vi "海洋光学光谱仪.vi"() -> ()   [LabVIEW 2018]
uses:
  <vilib>/Utility/file.llb/Write Delimited Spreadsheet (DBL).vi
  <vilib>/Utility/file.llb/Write Delimited Spreadsheet (string).vi
  Labview/SeaBreeze.lvlib
panel:
  in  "停止 2":bool
  out "当前时间":timestamp
  out "状态":string
  out "is Big Energy":bool
  out "time":string
  out "温度计":dbl(slide) scale=0.0..100.0
  out "湿度":dbl
  in  "VISA resource name":refnum<visa-resource-name>="COM3" caption="VISA资源名称"
  in  "停止":bool
  out "error_code out end":i32
  in  "count":dbl
  out "center2":dbl
  in  "baseline":dbl=2000.0 format="%#_13g"
  out "长度":i32
  out "center wavelength":dbl
  out "falling":dbl
  out "FPWM":dbl
  out "rasing":dbl
  in  "mode 触发模式为2":i32=2
  out "Type":string
  out "Grpah":cluster{"Y":dbl[], "Y":dbl[]}[](graph)
  out "Pixels":i32
  in  "integration time(us)":u32=60000
  out "Serial Number":string
  out "Found Spectrometer":string
  out "error_code out":i32
  in  "error_code":i32
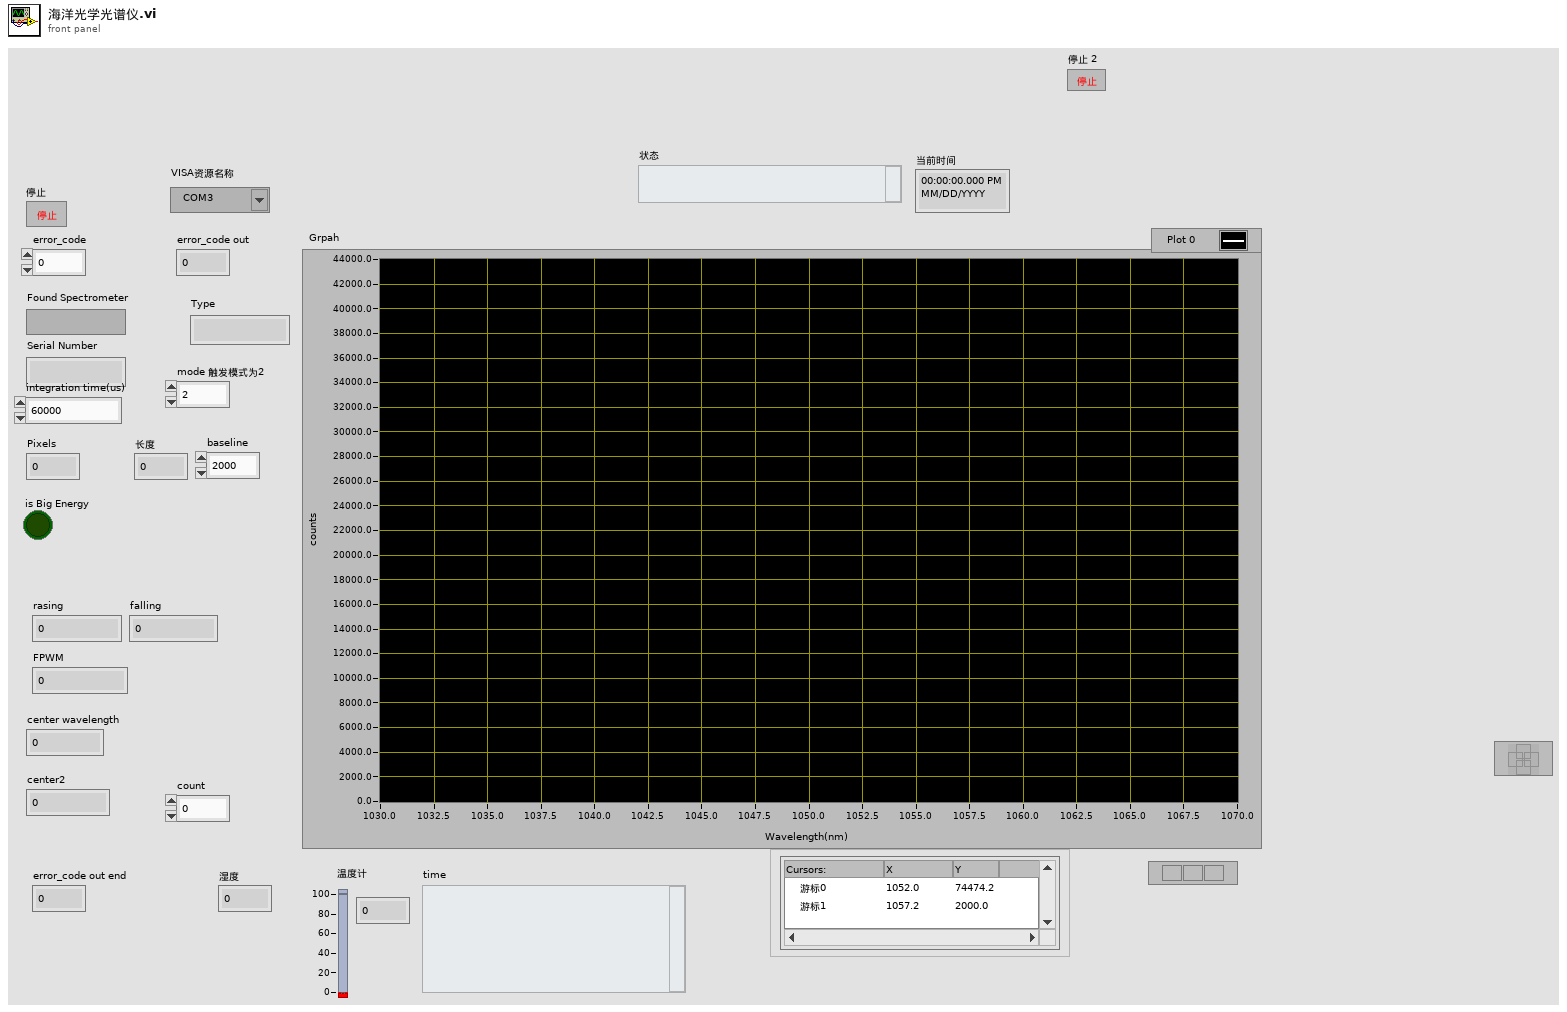
[diagram p1: front panel]
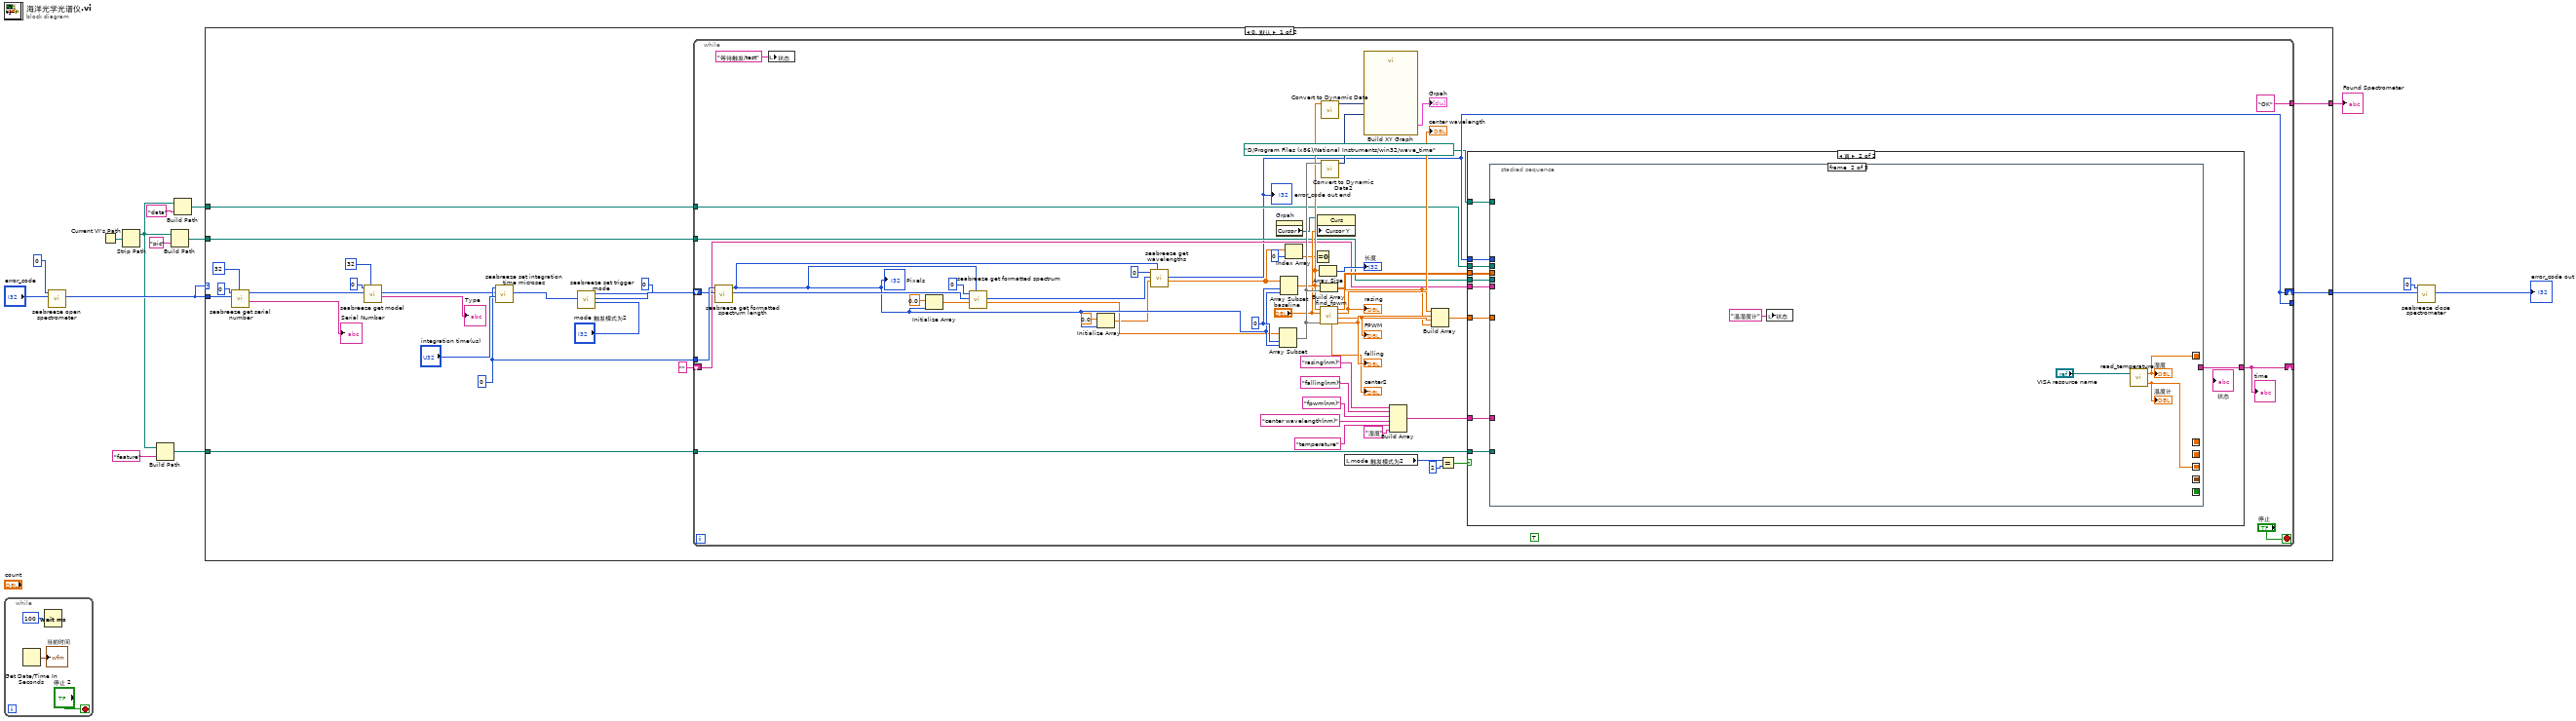
[diagram p0: block diagram]
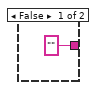
[diagram p2: hidden frame]
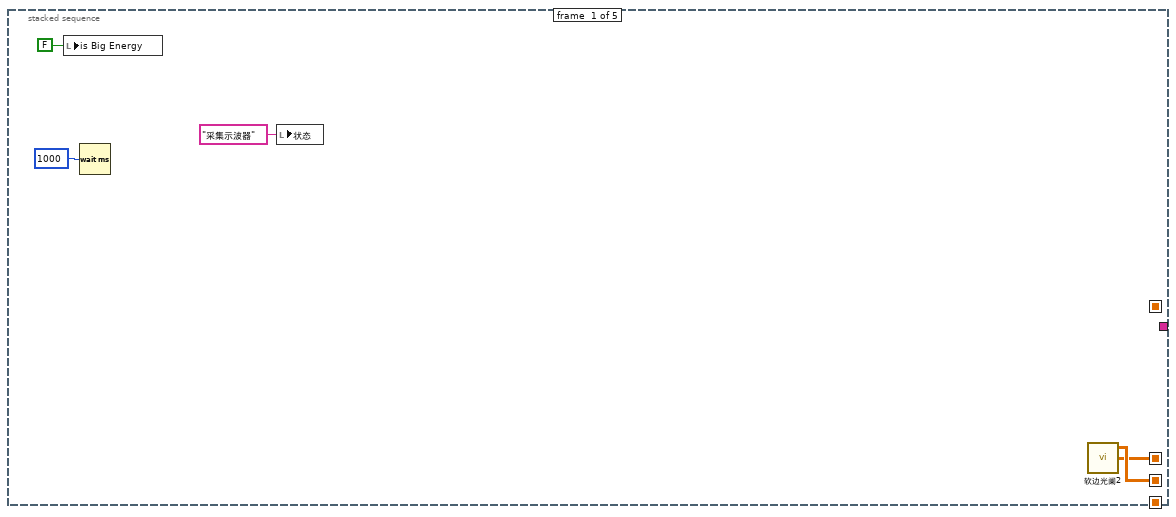
[diagram p3: hidden frame]
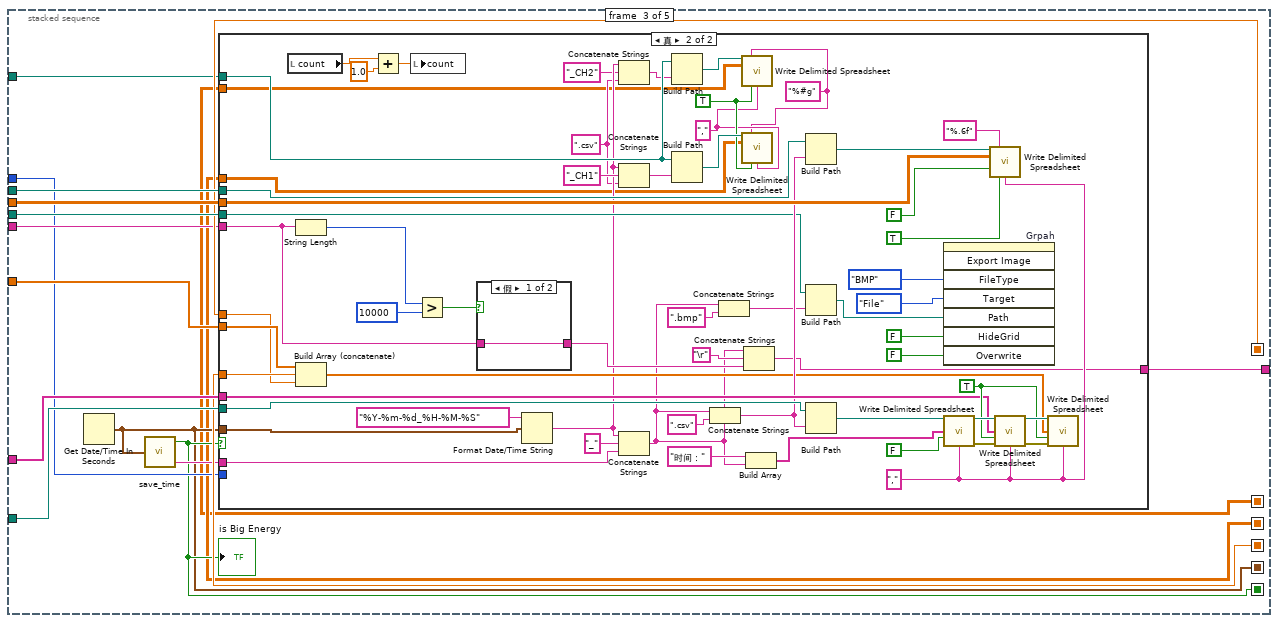
[diagram p4: hidden frame]
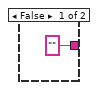
[diagram p5: hidden frame]
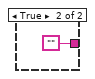
[diagram p6: hidden frame]
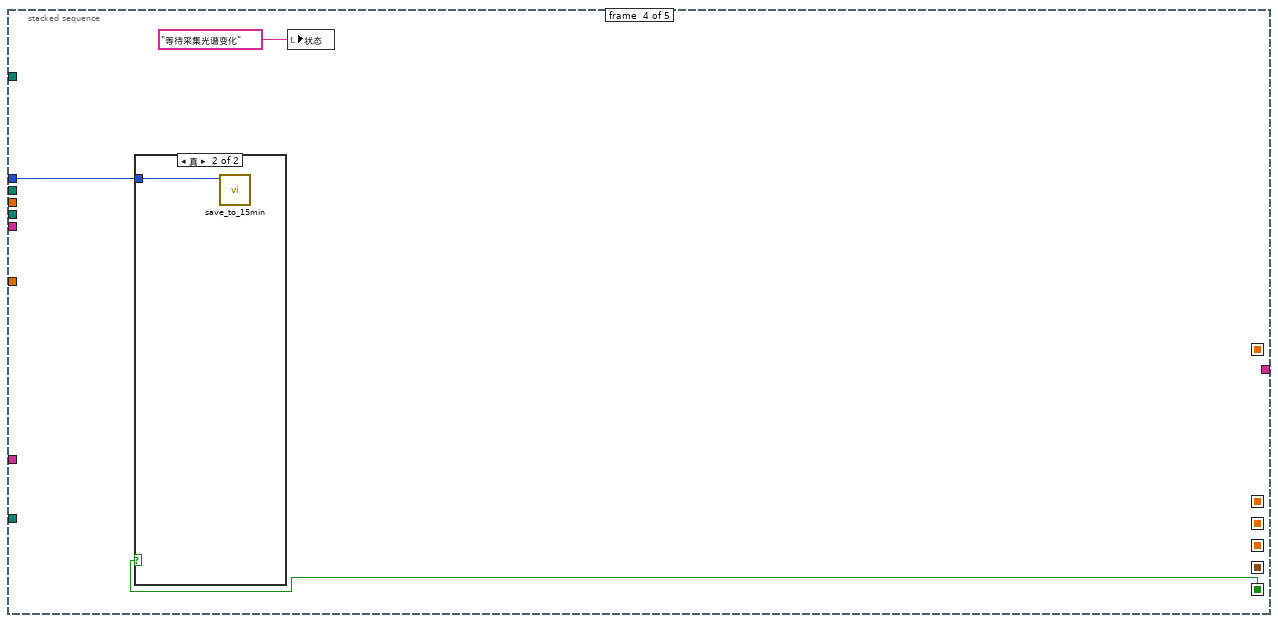
[diagram p7: hidden frame]
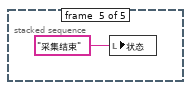
[diagram p9: hidden frame]
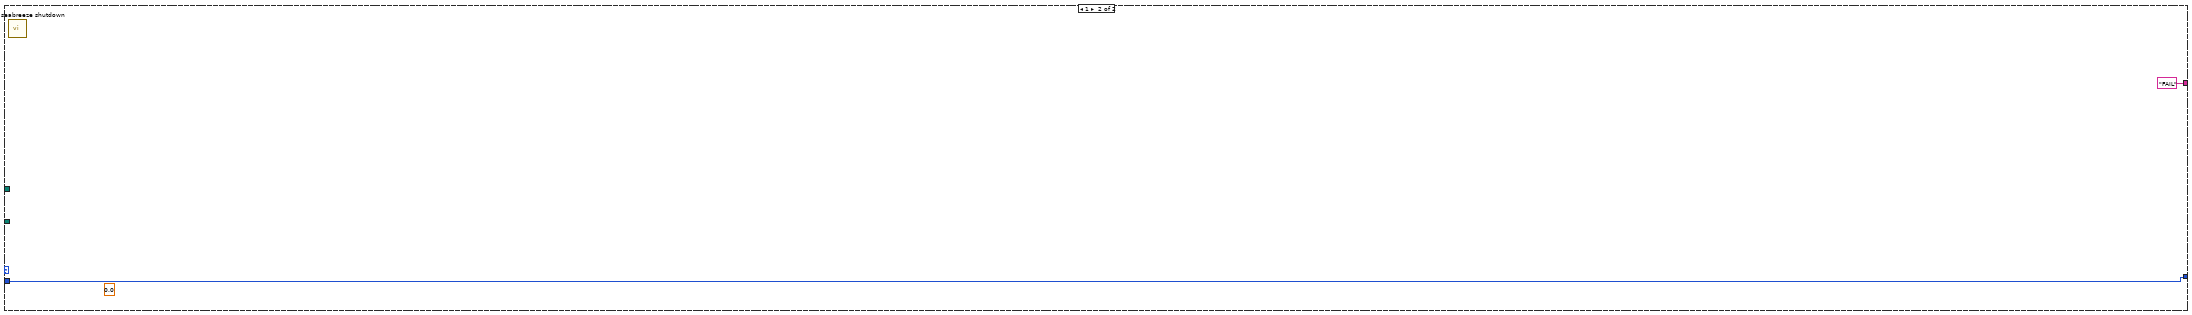
[diagram p10: hidden frame]
diagram:
  n1 = while {
    stop <- "停止 2" stop-if-true
    n2 = Get Date/Time In Seconds() -> (seconds since 1Jan1904=→"当前时间":timestamp)
    n3 = Wait (ms)(milliseconds to wait=u32 100 ("等待时间（毫秒）")) -> ()  [unwired: 1 out]
  }
  n4 = call "seabreeze open spectrometer.vi"("error_code"="error_code", "index"=0) -> ("error_code out"=w10:i32)  [unwired: 8 in, 1 out]
  n5 = Current VI's Path() -> (path=w8:path)
  n6 = Strip Path(path=w8) -> (stripped path=w3:path)  [unwired: 1 out]
  n7 = Build Path(base path=w3, name or relative path="feature" ("名称或相对路径")) -> (appended path=w4:path)
  n8 = Build Path(base path=w3, name or relative path="pic" ("名称或相对路径")) -> (appended path=w1:path)
  n9 = Build Path(base path=w3, name or relative path="data" ("名称或相对路径")) -> (appended path=w5:path)
  n10 = case shown="0, 默认" w10 {
    tunnel: [w39 "FAIL" ("Found Spectrometer")] -> w13
    tunnel: [w23 w197] -> w9
    tunnel: w10 -> [w24 w197]
    tunnel: w5 -> [w22 _]
    tunnel: w4 -> [w21 _]
    tunnel: w1 -> [w20 _]
    frame 0, Default {
      w34 = 0 ("index")
      n11 = call "seabreeze get serial number.vi"("buffer_length"=32, "error_code"=w24, "index"=0) -> ("buffer out"=→"Serial Number":string, "function return"=w30:i32)  [unwired: 6 in, 1 out]
      n12 = call "seabreeze get model.vi"("buffer_length"=32, "error_code"=w30, "index"=0) -> ("buffer out"=→"Type":string, "error_code out"=w29:i32)  [unwired: 6 in, 1 out]
      n13 = call "seabreeze set integration time microsec.vi"("integration_time_micros"="integration time(us)", "error_code"=w29, "index"=w34) -> ("error_code out"=w28:i32)  [unwired: 8 in]
      n14 = call "seabreeze set trigger mode.vi"("mode"="mode 触发模式为2", "error_code"=w28, "index"=0) -> ("error_code out"=w27:i32)  [unwired: 8 in]
      n15 = while {
        tunnel: ["OK" ("Found Spectrometer")] -> w39
        tunnel: w34 -> [w89]
        tunnel: [w42] -> _
        shift-right: [w42] -> w23
        shift-left: w27 -> [w81]
        tunnel: w22 -> [w49]
        tunnel: w21 -> [w48]
        tunnel: w20 -> [w47]
        shift-right: [w43] -> _
        shift-left: "" ("date/time string") -> [w44]
        stop <- "停止" stop-if-true
        (unwired) TRUE
        w68 = 0 ("索引")
        n16 = call "seabreeze get formatted spectrum length.vi"("error_code"=w81, "index"=w89) -> ("error_code out"=w88:i32, "function return"=w67:i32)  [unwired: 8 in]
        "Pixels" <- w67
        n17 = local write "状态"("等待触发/test") -> ()
        n18 = Initialize Array(0.0 ("element"), w67) -> (w57:dbl[])
        n19 = call "seabreeze get formatted spectrum.vi"("buffer_length"=w67, "buffer"=w57, "error_code"=w88, "index"=0) -> ("buffer out"=w61:dbl[], "error_code out"=w86:i32)  [unwired: 5 in, 1 out]
        n20 = Initialize Array(0.0 ("element"), w67) -> (w58:dbl[])
        n21 = call "seabreeze get wavelengths.vi"("length"=w67, "wavelengths"=w58, "error_code"=w86, "index"=0) -> ("wavelengths out"=w62:dbl[], "error_code out"=w42:i32)  [unwired: 5 in, 1 out]
        "error_code out end" <- w42
        n22 = property on="Grpah" class="XYGraph (严格)"() -> ("Cursor"=w64:refnum<vi>)  [unwired: 2 in, 2 out]
        n23 = Array Subset(array=w61, index=w68, length=w67) -> (w69:dbl[])
        n24 = Array Subset(array=w62, index=w68, length=w67) -> (w66:dbl[])
        n25 = Index Array(array=w62, index=0 ("索引")) -> (element=w59:dbl)
        n26 = Equal To 0?(x=w59) -> ()  [unwired: 1 out]
        n27 = property class="Curs"(reference=w64, "Cursor Y"="baseline") -> ()  [unwired: 1 in, 2 out]
        n28 = Array Size(array=w66) -> (size(s)=→"长度":i32)
        n29 = Build Array(w66, w69) -> (w56:dbl[][])
        n30 = call "find_fpwm.vi"("Y"=w69, "baseline"="baseline", "X"=w66) -> ("falling"=w74:dbl, "FPWM"=w73:dbl, "rasing"=w75:dbl, "center wavelength"=w71:dbl, "center2"=→"center2":dbl)  [unwired: 4 in]
        "rasing" <- w75
        "FPWM" <- w73
        "falling" <- w74
        "center wavelength" <- w71
        n31 = call "Convert to Dynamic Data"("Array"=w66) -> ("Dynamic Data Type"=w80:dynamicdata)  [unwired: 3 in]
        n32 = call "Convert to Dynamic Data2"("Array"=w69) -> ("Dynamic Data Type"=w79:dynamicdata)  [unwired: 3 in]
        n33 = local read "mode 触发模式为2"() -> (w52:i32)
        n34 = call "Build XY Graph"("Y Input"=w79, "X Input"=w80) -> ("XY Graph"=→"Grpah":cluster{"Y":dbl[], "Y":dbl[]}[])  [unwired: 3 in, 6 out]
        n35 = Build Array("rasing(nm)", "falling(nm)", "fpwm(nm)", "center wavelength(nm)", "temperature" ("元素"), "湿度" ("元素")) -> (w55:string[])
        n36 = Build Array(w75, w74, w73, w71) -> (w54:dbl[])
        n37 = Equal?(x=w52, y=2) -> (x = y?=w50:bool)
        n38 = case shown="真" w50 {
          tunnel: w56 -> [_ w101]
          tunnel: w55 -> [_ w100]
          tunnel: w54 -> [_ w99]
          tunnel: w49 -> [_ w98]
          tunnel: w48 -> [_ w97]
          tunnel: w47 -> [_ w96]
          tunnel: ["" w95] -> w43
          tunnel: w44 -> [_ w94]
          tunnel: w42 -> [_ w93]
          tunnel: path "D:/Program Files (x86)/National Instruments/win32/wave_time" ("Path") -> [_ w92]
          frame False {
          }
          frame True {
            n39 = stacked-sequence {
              seq-local: [_ w109 _ _ _] -> [_ _ w121 _ _]
              seq-local: [_ w108 _ _ _] -> [_ _ w120 _ _]
              seq-local: [_ _ w115 _ _] -> [_ _ _ w192 _]
              seq-local: [_ _ w114 _ _] -> [_ _ _ _ _]
              seq-local: [w106 _ _ _ _] -> [_ _ w112 _ _]
              seq-local: [w105 _ _ _ _] -> [_ _ w111 _ _]
              tunnel: w101 -> [_ _ w127 _ _]
              tunnel: w100 -> [_ _ w126 _ _]
              tunnel: w99 -> [_ _ w122 _ _]
              tunnel: w98 -> [_ _ w125 _ _]
              tunnel: w97 -> [_ _ w124 _ _]
              tunnel: w96 -> [_ _ w123 _ _]
              tunnel: [_ _ w119 _ _] -> w95
              tunnel: w94 -> [_ _ w118 _ _]
              tunnel: w93 -> [_ _ w116 w194 _]
              tunnel: w92 -> [_ _ w113 _ _]
              frame #0 {
                n40 = local write "is Big Energy"(FALSE) -> ()
                n41 = Wait (ms)(milliseconds to wait=u32 1000 ("等待时间（毫秒）")) -> ()  [unwired: 1 out]
                n42 = local write "状态"("采集示波器" ("状态")) -> ()
                n43 = call "软边光阑2.vi"() -> ("CH2"=w105:dbl[][], "CH1"=w106:dbl[][])  [unwired: 4 in, 1 out]
              }
              frame #1 {
                n44 = local write "状态"("温湿度计" ("状态")) -> ()
                n45 = call "read_temperature.vi"("VISA resource name"="VISA resource name") -> ("温度"=w109:dbl, "湿度"=w108:dbl)  [unwired: 1 in]
                "湿度" <- w108
                "温度计" <- w109
              }
              frame #2 {
                n46 = Get Date/Time In Seconds() -> (seconds since 1Jan1904=w114:timestamp)
                n47 = call "save_time.vi"("input time"=w114) -> ("Puls Width"=w117:string, "is Big Energy"=w115:bool)  [unwired: 2 in, 1 out]
                "is Big Energy" <- w115
                n48 = case shown="真" w115 {
                  tunnel: w127 -> [_ w185]
                  tunnel: w126 -> [_ w181]
                  tunnel: w125 -> [_ w176]
                  tunnel: w124 -> [_ w174]
                  tunnel: w123 -> [_ w163]
                  tunnel: w122 -> [_ w157]
                  tunnel: w121 -> [_ w156]
                  tunnel: w120 -> [_ w154]
                  tunnel: w114 -> [_ w153]
                  tunnel: ["" w151] -> w119
                  tunnel: w118 -> [_ w146]
                  tunnel: w117 -> [_ w143]
                  tunnel: w116 -> [_ _]
                  tunnel: w113 -> [_ w139]
                  tunnel: w112 -> [_ w131]
                  tunnel: w111 -> [_ w130]
                  frame False {
                  }
                  frame True {
                    w129 = "%#g" ("format (%.3f)")
                    w133 = "," ("delimiter (\\t)")
                    w134 = TRUE ("transpose? (no:F)")
                    w136 = ".csv" ("字符串")
                    w167 = "," ("delimiter (\\t)")
                    w182 = TRUE ("append to file? (new file:F)")
                    n49 = local read "count"() -> (w179:dbl)
                    n50 = String Length(string=w146) -> (length=w150:i32)
                    n51 = Build Array (concatenate)(w157, w156, w154) -> (w155:dbl[])
                    n52 = Add(x=w179, y=1.0) -> (x+y=w178:dbl)
                    n53 = local write "count"(w178) -> ()
                    n54 = Greater?(x=w150, y=10000) -> (0:w148:bool)
                    n55 = case shown="假" w148 {
                      tunnel: [w190 ""] -> w147
                      tunnel: w146 -> [w190 _]
                      frame False {
                      }
                      frame True {
                      }
                    }
                    n56 = Format Date/Time String(time format string (%c)="%Y-%m-%d_%H-%M-%S" ("时间格式字符串(%c)"), seconds (now)=w153) -> (date/time string=w138:string)  [unwired: 1 in]
                    n57 = Concatenate Strings(w138, "_CH2" ("字符串"), w136) -> (w135:string)
                    n58 = Concatenate Strings(w138, "_CH1" ("字符串"), w136) -> (w141:string)
                    n59 = Concatenate Strings(w138, "_" ("字符串"), w143) -> (w145:string)
                    n60 = Build Path(base path=w139, name or relative path=w135) -> (appended path=w132:path)
                    n61 = Build Path(base path=w139, name or relative path=w141) -> (appended path=w140:path)
                    n62 = Concatenate Strings(w145, ".csv" ("字符串")) -> (w168:string)
                    n63 = Concatenate Strings(w145, ".bmp" ("字符串")) -> (w164:string)
                    n64 = call-poly <vilib>:"Write Delimited Spreadsheet.vi"("file path (dialog if empty)"=w132, "format (%.3f)"=w129, "2D data"=w130, "transpose? (no:F)"=w134, "delimiter (\\t)"=w133) -> ()  [unwired: 9 in, 2 out]
                    n65 = call-poly <vilib>:"Write Delimited Spreadsheet.vi"("file path (dialog if empty)"=w140, "format (%.3f)"=w129, "2D data"=w131, "transpose? (no:F)"=w134, "delimiter (\\t)"=w133) -> ()  [unwired: 9 in, 2 out]
                    n66 = Concatenate Strings(w145, "\r", w147) -> (w151:string)
                    n67 = Build Array("时间：" ("元素"), w145) -> (w170:string[])
                    n68 = Build Path(base path=w176, name or relative path=w168) -> (appended path=w175:path)
                    n69 = Build Path(base path=w163, name or relative path=w164) -> (appended path=w160:path)
                    n70 = Build Path(base path=w174, name or relative path=w168) -> (appended path=w173:path)
                    n71 = invoke on="Grpah" class="XYGraph (严格)" method="Export Image"("FileType"=enum32{"BMP", "EPS", "EMF", "PICT"}."BMP" ("文件类型"), "Target"=enum32{"File", "Clipboard"}."File" ("目标"), "Path"=w160, "HideGrid"=FALSE ("隐藏网格"), "Overwrite"=FALSE ("始终覆盖")) -> ()  [unwired: 3 in, 8 out]
                    n72 = call-poly <vilib>:"Write Delimited Spreadsheet.vi"("file path (dialog if empty)"=w173, "1D data"=w170, "append to file? (new file:F)"=FALSE, "delimiter (\\t)"=w167) -> ("new file path (Not A Path if cancelled)"=w189:path, "error out"=w188:errorcluster)  [unwired: 10 in]
                    n73 = call-poly <vilib>:"Write Delimited Spreadsheet.vi"("file path (dialog if empty)"=w175, "format (%.3f)"="%.6f", "2D data"=w185, "append to file? (new file:F)"=FALSE, "transpose? (no:F)"=TRUE, "delimiter (\\t)"=w167) -> ()  [unwired: 8 in, 2 out]
                    n74 = call-poly <vilib>:"Write Delimited Spreadsheet.vi"("file path (dialog if empty)"=w189, "1D data"=w181, "append to file? (new file:F)"=w182, "error in (no error)"=w188, "delimiter (\\t)"=w167) -> ("new file path (Not A Path if cancelled)"=w186:path, "error out"=w187:errorcluster)  [unwired: 9 in]
                    n75 = call-poly <vilib>:"Write Delimited Spreadsheet.vi"("file path (dialog if empty)"=w186, "1D data"=w155, "append to file? (new file:F)"=w182, "error in (no error)"=w187, "delimiter (\\t)"=w167) -> ()  [unwired: 9 in, 2 out]
                  }
                }
              }
              frame #3 {
                n76 = case shown="真" w192 {
                  tunnel: w194 -> [_ w195]
                  frame False {
                  }
                  frame True {
                    n77 = call "save_to_15min.vi"("error_code"=w195) -> ()  [unwired: 11 in]
                  }
                }
                n78 = local write "状态"("等待采集光谱变化") -> ()
              }
              frame #4 {
                n79 = local write "状态"("采集结束") -> ()
              }
            }
          }
        }
        "time" <- w43
      }
    }
    frame 1 {
      (unwired) 0.0
      n80 = call "seabreeze shutdown.vi"() -> ()  [unwired: 12 in]
    }
  }
  "Found Spectrometer" <- w13
  n81 = call "seabreeze close spectrometer.vi"("error_code"=w9, "index"=0) -> ("error_code out"=→"error_code out":i32)  [unwired: 8 in, 1 out]
